vi "Extract_Images_From_CIFAR10.vi"(6 "Labels":string[](array[string]), 7 "File Names":string[](array[string])=["data_batch_1.bin", "data_batch_2.bin", "data_batch_3.bin", "data_batch_4.bin", "data_batch_5.bin"], 8 "error in":errorcluster, 10 "Destination Folder Path":path=path "D:/cifar-10-images/train", 11 "CIFAR Path":path=path "D:/cifar-10-batches-bin/train") -> (0 "error out":errorcluster)   [LabVIEW 2020]
panel:
  out "Progress":i32
  out "Total no of Images":i32
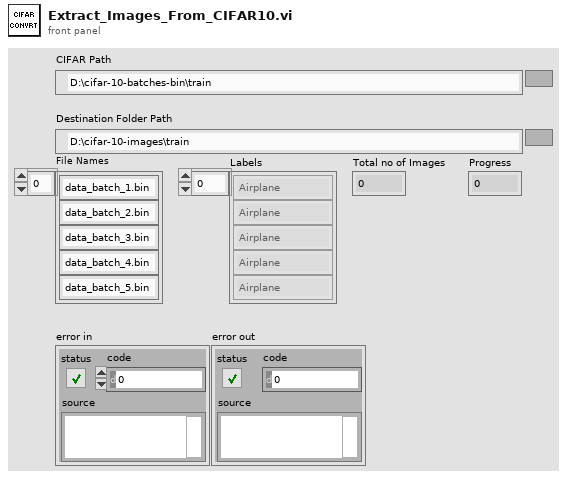
[diagram p1: front panel]
types:
  T1 = typedef "Image Type" = u32
  T2 = typedef "IMAQ Image.ctl" = refnum<image>
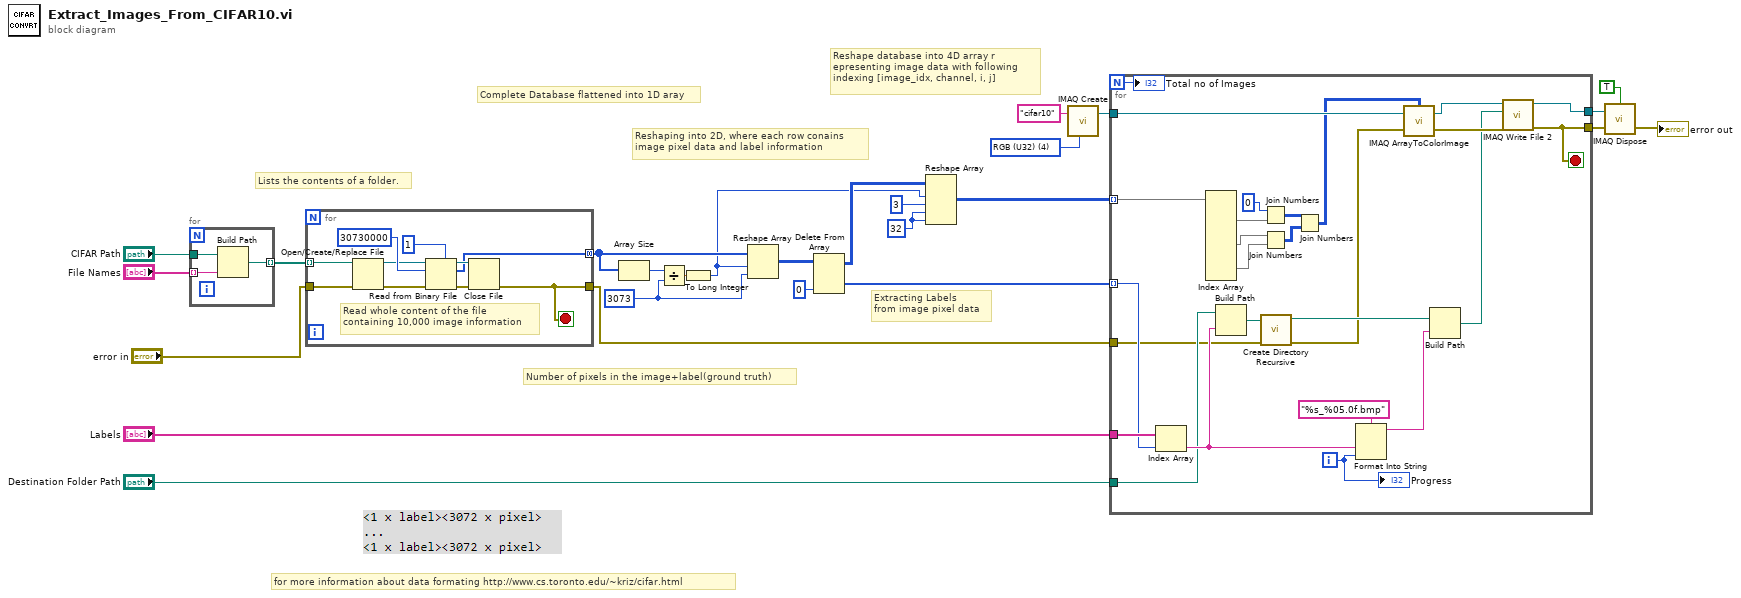
[diagram p0: block diagram]
diagram:
  w14 = T1 4 items=["Grayscale (U8)", "Grayscale (I16)", "Grayscale (SGL)", "Complex (CSG)", "RGB (U32)", "HSL (U32)", "RGB (U64)", "Grayscale (U16)"] ("Image Type")
  w17 = 32 ("dimension size")
  w20 = 3073 ("dimension size")
  # "for more information about data formating http://www.cs.toronto.edu/~kriz/cifar.html"
  # "Number of pixels in the image+label(ground truth)"
  # "Extracting Labels \nfrom image pixel data"
  # "Reshaping into 2D, where each row conains \nimage pixel data and label information"
  # "Reshape database into 4D array r\nepresenting image data with following \nindexing [image_idx, channel, i, j]"
  # "Complete Database flattened into 1D aray"
  # "Lists the contents of a folder."
  n1 = for {
    tunnel: "File Names" -> [w29] mode=indexing
    tunnel: "CIFAR Path" -> [w28]
    tunnel: [w27] -> w6 mode=indexing
    n2 = Build Path(base path=w28, name or relative path=w29) -> (appended path=w27:path)
  }
  n3 = for {
    tunnel: w6 -> [w39] mode=indexing
    tunnel: [w32] -> w22 mode=concatenating
    tunnel: [w30] -> w3
    tunnel: "error in" -> [w31]
    stop <- w30 stop-if-true
    # "Read whole content of the file\ncontaining 10,000 image information"
    n4 = Open/Create/Replace File(file path (use dialog)=w39, error in=w31) -> (refnum out=w35:refnum<file>, error out=w34:errorcluster)  [unwired: 4 in, 1 out]
    n5 = Read from Binary File(5:u8 1 ("y"), 8:w34, 10:30730000 ("count (1)"), 11:w35) -> (0:w37:errorcluster, 2:w32:u8[], 3:w36:refnum<file>)  [unwired: 2 in, 1 out]
    n6 = Close File(refnum=w36, error in=w37) -> (error out=w30:errorcluster)  [unwired: 1 out]
  }
  n7 = Array Size(array=w22) -> (size(s)=w21:i32)
  n8 = Divide(x=w21, y=w20) -> (x/y=w19:dbl)
  n9 = To Long Integer(number=w19) -> (32bit integer=w18:i32)
  n10 = Reshape Array(w22, w18, w20) -> (w23:u8[][])
  n11 = Delete From Array(array=w23, index (col)=0 ("disabled index (col)")) -> (deleted portion=w12:u8[], array with subset deleted=w24:u8[][])  [unwired: 2 in]
  n12 = Reshape Array(w24, w18, 3 ("dimension size"), w17, w17) -> (w13:u8[][][][])
  n13 = call "IMAQ Create"("Image Name"="cifar10", "Image Type"=w14) -> ("New Image"=w15:T2)  [unwired: 3 in, 1 out]
  n14 = for {
    N -> [w48]
    tunnel: w13 -> [w65] mode=indexing
    tunnel: w15 -> [w64]
    tunnel: w12 -> [w44] mode=indexing
    tunnel: [w40] -> w11
    tunnel: [w50] -> w10
    tunnel: "Labels" -> [w45]
    tunnel: "Destination Folder Path" -> [w42]
    tunnel: w3 -> [w41]
    i -> [w53]
    stop <- w40 stop-if-true
    n15 = Index Array(array=w45, index=w44) -> (element=w43:string)
    n16 = Index Array(array=w65) -> (element #1=w60:u8[][], element #2=w59:u8[][], element #3=w58:u8[][])  [unwired: 9 in]
    n17 = Build Path(base path=w42, name or relative path=w43) -> (appended path=w52:path)
    n18 = Join Numbers(hi=u8 0, lo=w60) -> ((hi.lo)=w63:u16[][])
    n19 = Join Numbers(hi=w59, lo=w58) -> ((hi.lo)=w62:u16[][])
    n20 = call <vilib>:"Create Directory Recursive.vi"("error in (no error)"=w41, "directory"=w52) -> ("error out"=w49:errorcluster, "directory copy"=w51:path)  [unwired: 3 in, 1 out]
    n21 = Join Numbers(hi=w63, lo=w62) -> ((hi.lo)=w61:u32[][])
    n22 = Format Into String(format string="%s_%05.0f.bmp", w43, w53) -> (resulting string=w46:string)  [unwired: 2 in, 1 out]
    n23 = call "IMAQ ArrayToColorImage"("Image Pixels (U32)"=w61, "Image"=w64, "error in (no error)"=w49) -> ("Image Out"=w56:T2, "error out"=w57:errorcluster)  [unwired: 2 in]
    n24 = Build Path(base path=w51, name or relative path=w46) -> (appended path=w55:path)
    n25 = call-poly "IMAQ Write File 2"("error in (no error)"=w57, "File Path"=w55, "Image"=w56) -> ("error out"=w40:errorcluster, "Image Out (duplicate)"=w50:T2)  [unwired: 7 in]
    "Total no of Images" <- w48
    "Progress" <- w53
  }
  n26 = call "IMAQ Dispose"("All Images? (No)"=TRUE, "Image"=w10, "error in (no error)"=w11) -> ("error out"=→"error out":errorcluster)  [unwired: 3 in]
